vi "BinSearchVIhotcold.vi"(6 "RN":sgl, 8 "X0":sgl=0.5, 11 "Ring":i16(ring) items=["Cold", "Warm", "Hot"]) -> (3 "Xpot":sgl)   [LabVIEW 2019]
uses:
  <vilib>/Platform/TimedLoop/XDataNode/timing_clust.ctl
  <vilib>/Platform/TimedLoop/XDataNode/nitl_modes.ctl
  <vilib>/Platform/TimedLoop/XDataNode/wakeup.ctl
  <vilib>/rvi/Emulation/niFpgaGetClockAttributes.vi
  <vilib>/rvi/Emulation/niFpgaSctlEmulationGetInTimedLoop.vi
  <vilib>/rvi/Emulation/niFpgaEmulationReportErrorSimple.vi
  <vilib>/rvi/Emulation/niFpgaCriticalErrorInLSC.vi
  <vilib>/Platform/TimedLoop/XDataNode/XDataNode.xnode
  <vilib>/Platform/TimedLoop/XDataNode/XDNodeRunTimeDep.lvlib
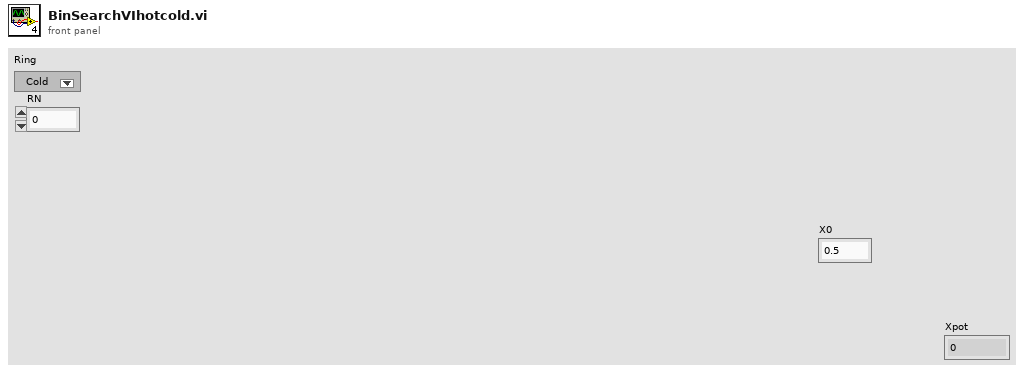
[diagram p1: front panel]
types:
  T1 = typedef "XDNodeRunTimeDep.lvlib/timing_clust.ctl" = cluster{"Expected End [f-1]":u64, "Actual End [f-1]":u64, "Finished Late? [f-1]":bool, "Expected End [i-1]":u64, "Actual End [i-1]":u64, "Finished Late? [i-1]":bool, "Expected Start [i]":u64, "Actual Start [i]":u64, "Expected Start [f]":u64, "Actual Start [f]":u64, "Source Name":string, "Structure Name":string, "Period":i64, "Deadline":i64, "Offset":i64, "Start":i64, "Priority":i32, "Timeout":i32, "Mode":T2, "Wakeup Reason":T3, "Error":errorcluster, "Source Type":string, "Secondary Source Type":string, "Global End Time":u64, "Global Start Time":u64, "Frame Duration":u64, "Iteration Duration":u64, "Assigned CPU":i32, "I/O Scan Engine Mode":u32}
  T2 = typedef "XDNodeRunTimeDep.lvlib/nitl_modes.ctl" = enum32{"No Change", "Process missed periods, maintain original phase", "Discard missed periods, maintain original phase", "Process missed periods, ignore original phase", "Discard missed periods, ignore original phase"}
  T3 = typedef "XDNodeRunTimeDep.lvlib/wakeup.ctl" = enum32{"Normal", "Aborted", "Asynchronous wakeup", "Timing source error", "Timed loop error", "Timeout"}
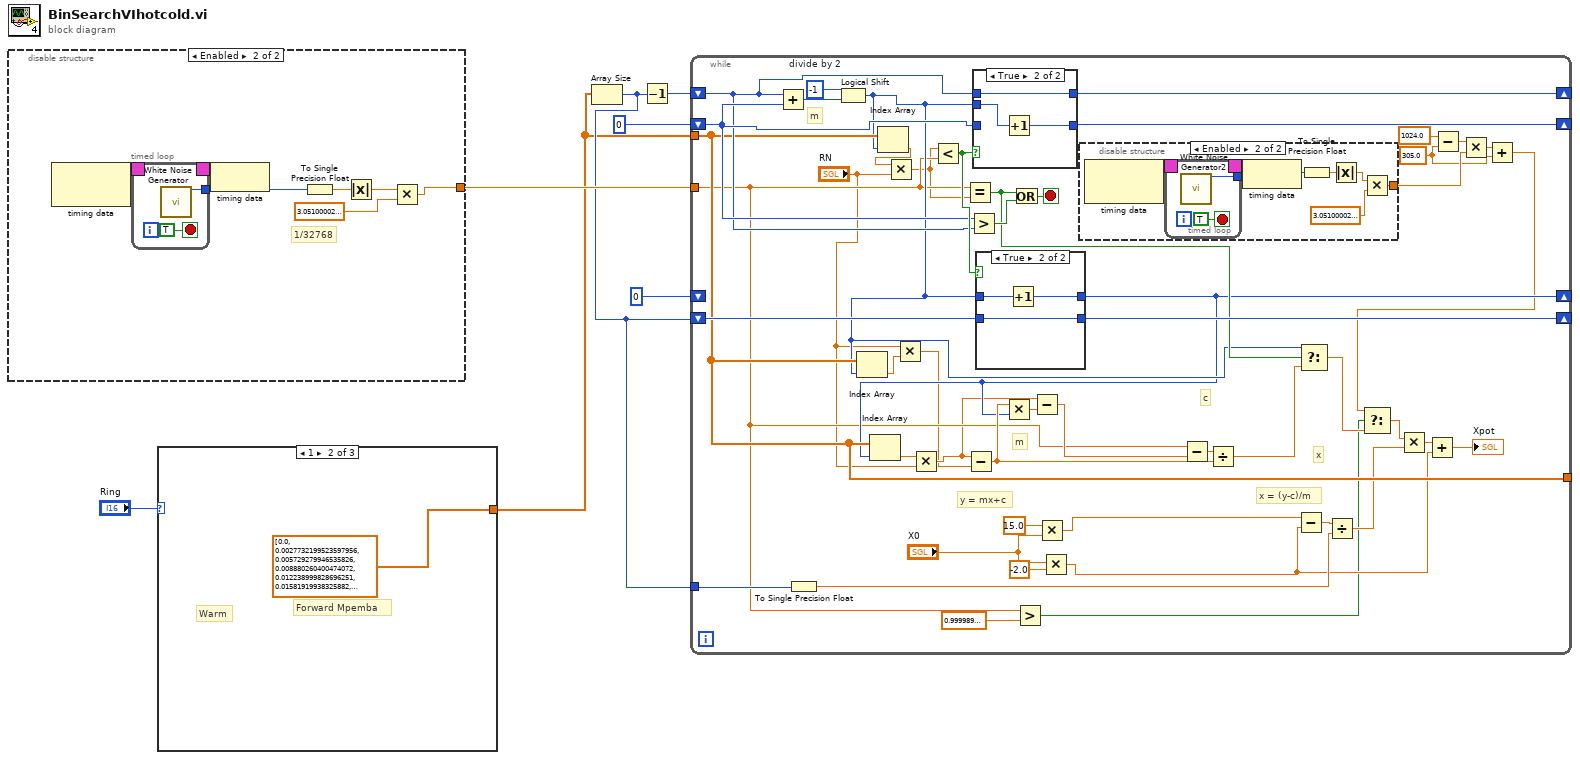
[diagram p0: block diagram]
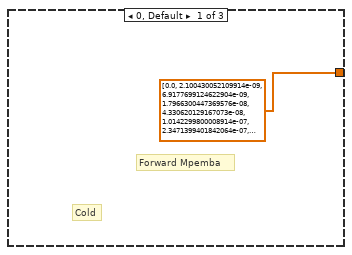
[diagram p2: hidden frame]
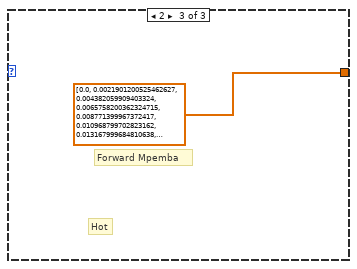
[diagram p3: hidden frame]
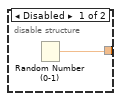
[diagram p4: hidden frame]
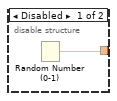
[diagram p5: hidden frame]
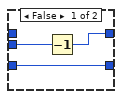
[diagram p7: hidden frame]
diagram:
  n1 = disable-structure shown="Enabled" {
    disable-tunnel: [w8 w11] -> w4
    frame Disabled {
      n2 = Random Number (0-1)() -> (number: 0 to 1=w8:dbl)
    }
    frame Enabled {
      # "1/32768"
      n3 = node-c288() -> (w10:T1)  [unwired: 1 in]
      n4 = timed-loop {
        timing: w10 -> [_]
        timing-out: [_] -> w9
        tunnel: [w17] -> w15
        stop <- TRUE stop-if-true
        n5 = call "White Noise Generator"() -> ("white noise out"=w17:i16)  [unwired: 15 in]
      }
      n6 = node-c288(w9) -> ()
      n7 = To Single Precision Float(number=w15) -> (single precision float=w13:sgl)
      n8 = Absolute Value(x=w13) -> (abs(x)=w12:sgl)
      n9 = Multiply(x=w12, y=sgl 3.051e-05) -> (x*y=w11:sgl)
    }
  }
  n10 = case shown="1" "Ring" {
    tunnel: [sgl[] [0.0, 2.10043e-09, 6.91777e-09, 1.79663e-08, 4.33062e-08, 1.01423e-07, 2.34714e-07, 5.40417e-07, 1.24154e-06, 2.84958e-06, 6.60417e-06, 1.50495e-05, 3.29051e-05, 6.8487e-05, 0.000135501, 0.0002551, 0.000457891, 0.000785411, 0.0012905, 0.00203611, 0.00309218, 0.00453075, 0.00641965, 0.00881572, 0.0117584, 0.0152648, 0.019327, 0.0239115, 0.0289619, 0.0344029, 0.0401462, 0.0460966, 0.0521583, 0.0582401, 0.0642597, 0.0701466, 0.0758436, 0.0813074, 0.0865076, 0.0914259, 0.0960546, 0.100394, 0.104453, 0.108243, 0.11178, 0.115085, 0.118176, 0.121075, 0.123802, 0.126379, 0.128825, 0.13116, 0.133402, 0.135569, 0.137679, 0.139748, 0.141793, 0.143832, 0.14588, 0.147957, 0.150081, 0.152272, 0.154553, 0.156947, 0.159484, 0.162193, 0.165111, 0.16828, 0.171747, 0.175568, 0.179807, 0.184542, 0.189859, 0.195861, 0.202666, 0.210409, 0.219246, 0.229351, 0.240917, 0.254157, 0.269299, 0.286581, 0.306242, 0.32851, 0.353589, 0.381636, 0.412741, 0.446898, 0.483987, 0.523744, 0.565749, 0.609418, 0.654015, 0.698674, 0.742448, 0.784365, 0.823503, 0.859064, 0.890444, 0.917278, 0.939468, 0.957175, 0.970777, 0.980814, 0.987911, 0.992708, 0.9958, 0.997696, 0.998798, 0.999405, 0.99972, 0.999874, 0.999945, 0.999976, 0.999989, 0.999995, 0.999998, 0.999999, 0.999999, 0.999999, 1.0, 1.0, 1.0, 1.0, 1.0, 1.0, 1.0, 1.0, 1.0, 1.0, 1.0, 1.0, 1.0, 1.0, 1.0, 1.0, 1.0, 1.0, 1.0, 1.0, 1.0, 1.0, 1.0, 1.0, 1.0, 1.0, 1.0, 1.0, 1.0, 1.0, 1.0, 1.0, 1.0, 1.0, 1.0, 1.0, 1.0, 1.0, 1.0, 1.0, 1.0, 1.0, 1.0, 1.0, 1.0, 1.0, 1.0, 1.0, 1.0, 1.0, 1.0, 1.0, 1.0, 1.0, 1.0, 1.0, 1.0, 1.0, 1.0, 1.0, 1.0, 1.0, 1.0, 1.0, 1.0, 1.0, 1.0, 1.0, 1.0, 1.0, 1.0, 1.0, 1.0, 1.0, 1.0, 1.0, 1.0, 1.0, 1.0, 1.0, 1.0, 1.0, 1.0, 1.0, 1.0, 1.0, 1.0, 1.0, 1.0, 1.0, 1.0, 1.0, 1.0, 1.0, 1.0, 1.0, 1.0, 1.0, 1.0, 1.0, 1.0, 1.0, 1.0, 1.0, 1.0, 1.0, 1.0, 1.0, 1.0, 1.0, 1.0, 1.0, 1.0, 1.0, 1.0, 1.0, 1.0, 1.0, 1.0, 1.0, 1.0, 1.0, 1.0, 1.0, 1.0, 1.0, 1.0, 1.0, 1.0, 1.0, 1.0, 1.0, 1.0, 1.0, 1.0, 1.0, 1.0, 1.0, 1.0, 1.0, 1.0, 1.0, 1.0, 1.0, 1.0, 1.0, 1.0, 1.0, 1.0, 1.0, 1.0, 1.0, 1.0, 1.0, 1.0, 1.0, 1.0, 1.0, 1.0, 1.0, 1.0, 1.0, 1.0, 1.0, 1.0, 1.0, 1.0, 1.0, 1.0, 1.0, 1.0, 1.0, 1.0, 1.0, 1.0, 1.0, 1.0, 1.0, 1.0, 1.0, 1.0, 1.0, 1.0, 1.0, 1.0, 1.0, 1.0, 1.0, 1.0, 1.0, 1.0, 1.0, 1.0, 1.0, 1.0, 1.0, 1.0, 1.0, 1.0, 1.0, 1.0, 1.0, 1.0, 1.0, 1.0, 1.0, 1.0, 1.0, 1.0, 1.0, 1.0, 1.0, 1.0, 1.0, 1.0, 1.0, 1.0, 1.0, 1.0, 1.0, 1.0, 1.0, 1.0, 1.0, 1.0, 1.0, 1.0, 1.0, 1.0, 1.0, 1.0, 1.0, 1.0, 1.0, 1.0, 1.0, 1.0, 1.0, 1.0, 1.0, 1.0, 1.0, 1.0, 1.0, 1.0, 1.0, 1.0, 1.0, 1.0, 1.0, 1.0, 1.0, 1.0, 1.0, 1.0, 1.0, 1.0, 1.0, 1.0, 1.0, 1.0, 1.0, 1.0, 1.0, 1.0, 1.0, 1.0, 1.0, 1.0, 1.0, 1.0, 1.0, 1.0, 1.0, 1.0, 1.0, 1.0, 1.0, 1.0, 1.0, 1.0, 1.0, 1.0, 1.0, 1.0, 1.0, 1.0, 1.0, 1.0, 1.0, 1.0, 1.0, 1.0, 1.0, 1.0, 1.0, 1.0, 1.0, 1.0, 1.0, 1.0, 1.0, 1.0, 1.0, 1.0, 1.0, 1.0, 1.0, 1.0, 1.0, 1.0, 1.0, 1.0, 1.0, 1.0, 1.0, 1.0, 1.0, 1.0, 1.0, 1.0, 1.0, 1.0, 1.0, 1.0, 1.0, 1.0, 1.0, 1.0, 1.0, 1.0, 1.0, 1.0, 1.0, 1.0, 1.0, 1.0, 1.0, 1.0, 1.0, 1.0, 1.0, 1.0, 1.0, 1.0, 1.0, 1.0, 1.0, 1.0, 1.0, 1.0, 1.0, 1.0, 1.0, 1.0, 1.0, 1.0, 1.0, 1.0, 1.0, 1.0, 1.0, 1.0, 1.0, 1.0, 1.0, 1.0, 1.0, 1.0, 1.0, 1.0, 1.0, 1.0, 1.0, 1.0, 1.0, 1.0, 1.0, 1.0, 1.0, 1.0, 1.0, 1.0, 1.0, 1.0, 1.0, 1.0, 1.0, 1.0, 1.0, 1.0, 1.0] ("Init Data Out") sgl[] [0.0, 0.00277322, 0.00572928, 0.00888026, 0.012239, 0.0158192, 0.0196354, 0.0237033, 0.0280394, 0.0326614, 0.0375931, 0.0428469, 0.0484165, 0.0542936, 0.0604679, 0.0669269, 0.0736569, 0.0806426, 0.0878674, 0.0953142, 0.102965, 0.110802, 0.118805, 0.126958, 0.135242, 0.143639, 0.152132, 0.160705, 0.169342, 0.178029, 0.186753, 0.1955, 0.20426, 0.213023, 0.221778, 0.230518, 0.239236, 0.247927, 0.256584, 0.265204, 0.273784, 0.282321, 0.290814, 0.299263, 0.307668, 0.316028, 0.324345, 0.332622, 0.34086, 0.349062, 0.357231, 0.365371, 0.373486, 0.381579, 0.389656, 0.397721, 0.405778, 0.413834, 0.421893, 0.42996, 0.438041, 0.446141, 0.454267, 0.462422, 0.470614, 0.478848, 0.487129, 0.495462, 0.503852, 0.512306, 0.520828, 0.529422, 0.538093, 0.546845, 0.555682, 0.564607, 0.573624, 0.582733, 0.591938, 0.60124, 0.610637, 0.620131, 0.629719, 0.6394, 0.64917, 0.659025, 0.668958, 0.678964, 0.689033, 0.699156, 0.709323, 0.71952, 0.729733, 0.739948, 0.750147, 0.760311, 0.770422, 0.780458, 0.790398, 0.800217, 0.809893, 0.819401, 0.828716, 0.837814, 0.84667, 0.85526, 0.863562, 0.871554, 0.879215, 0.886528, 0.893477, 0.900049, 0.906232, 0.912032, 0.917473, 0.922578, 0.927367, 0.93186, 0.936075, 0.940029, 0.943739, 0.947219, 0.950484, 0.953547, 0.95642, 0.959116, 0.961645, 0.964018, 0.966243, 0.968332, 0.97029, 0.972128, 0.973852, 0.97547, 0.976987, 0.978411, 0.979746, 0.980999, 0.982175, 0.983277, 0.984312, 0.985282, 0.986193, 0.987047, 0.987848, 0.9886, 0.989305, 0.989967, 0.990587, 0.99117, 0.991716, 0.992228, 0.992709, 0.99316, 0.993583, 0.99398, 0.994353, 0.994702, 0.99503, 0.995337, 0.995626, 0.995897, 0.99615, 0.996389, 0.996612, 0.996822, 0.997018, 0.997203, 0.997376, 0.997538, 0.997691, 0.997834, 0.997968, 0.998093, 0.998211, 0.998322, 0.998426, 0.998523, 0.998615, 0.9987, 0.998781, 0.998856, 0.998927, 0.998994, 0.999056, 0.999114, 0.999169, 0.999221, 0.999269, 0.999314, 0.999357, 0.999397, 0.999434, 0.999469, 0.999502, 0.999533, 0.999562, 0.999589, 0.999614, 0.999638, 0.999661, 0.999682, 0.999702, 0.99972, 0.999738, 0.999754, 0.999769, 0.999783, 0.999797, 0.99981, 0.999821, 0.999833, 0.999843, 0.999853, 0.999862, 0.99987, 0.999879, 0.999886, 0.999893, 0.9999, 0.999906, 0.999912, 0.999917, 0.999923, 0.999927, 0.999932, 0.999936, 0.99994, 0.999944, 0.999948, 0.999951, 0.999954, 0.999957, 0.99996, 0.999962, 0.999965, 0.999967, 0.999969, 0.999971, 0.999973, 0.999974, 0.999976, 0.999978, 0.999979, 0.99998, 0.999982, 0.999983, 0.999984, 0.999985, 0.999986, 0.999987, 0.999988, 0.999989, 0.999989, 0.99999, 0.999991, 0.999991, 0.999992, 0.999992, 0.999993, 0.999994, 0.999994, 0.999994, 0.999995, 0.999995, 0.999996, 0.999996, 0.999996, 0.999996, 0.999997, 0.999997, 0.999997, 0.999997, 0.999998, 0.999998, 0.999998, 0.999998, 0.999998, 0.999999, 0.999999, 0.999999, 0.999999, 0.999999, 0.999999, 0.999999, 0.999999, 1.0, 1.0, 1.0, 1.0, 1.0, 1.0, 1.0, 1.0, 1.0, 1.0, 1.0, 1.0, 1.0, 1.0, 1.0, 1.0, 1.0, 1.0, 1.0, 1.0, 1.0, 1.0, 1.0, 1.0, 1.0, 1.0, 1.0, 1.0, 1.0, 1.0, 1.0, 1.0, 1.0, 1.0, 1.0, 1.0, 1.0, 1.0, 1.0, 1.0, 1.0, 1.0, 1.0, 1.0, 1.0, 1.0, 1.0, 1.0, 1.0, 1.0, 1.0, 1.0, 1.0, 1.0, 1.0, 1.0, 1.0, 1.0, 1.0, 1.0, 1.0, 1.0, 1.0, 1.0, 1.0, 1.0, 1.0, 1.0, 1.0, 1.0, 1.0, 1.0, 1.0, 1.0, 1.0, 1.0, 1.0, 1.0, 1.0, 1.0, 1.0, 1.0, 1.0, 1.0, 1.0, 1.0, 1.0, 1.0, 1.0, 1.0, 1.0, 1.0, 1.0, 1.0, 1.0, 1.0, 1.0, 1.0, 1.0, 1.0, 1.0, 1.0, 1.0, 1.0, 1.0, 1.0, 1.0, 1.0, 1.0, 1.0, 1.0, 1.0, 1.0, 1.0, 1.0, 1.0, 1.0, 1.0, 1.0, 1.0, 1.0, 1.0, 1.0, 1.0, 1.0, 1.0, 1.0, 1.0, 1.0, 1.0, 1.0, 1.0, 1.0, 1.0, 1.0, 1.0, 1.0, 1.0, 1.0, 1.0, 1.0, 1.0, 1.0, 1.0, 1.0, 1.0, 1.0, 1.0, 1.0, 1.0, 1.0, 1.0, 1.0, 1.0, 1.0, 1.0, 1.0, 1.0, 1.0, 1.0, 1.0, 1.0, 1.0, 1.0, 1.0, 1.0, 1.0, 1.0, 1.0, 1.0, 1.0, 1.0, 1.0, 1.0, 1.0, 1.0, 1.0, 1.0, 1.0, 1.0, 1.0, 1.0, 1.0, 1.0, 1.0, 1.0, 1.0, 1.0, 1.0, 1.0, 1.0, 1.0, 1.0, 1.0, 1.0, 1.0, 1.0, 1.0, 1.0, 1.0, 1.0, 1.0, 1.0, 1.0, 1.0, 1.0, 1.0, 1.0, 1.0, 1.0, 1.0, 1.0, 1.0, 1.0, 1.0, 1.0, 1.0, 1.0, 1.0, 1.0, 1.0, 1.0, 1.0, 1.0, 1.0, 1.0] ("Init Data Out") sgl[] [0.0, 0.00219012, 0.00438206, 0.00657582, 0.0087714, 0.0109688, 0.013168, 0.0153691, 0.017572, 0.0197767, 0.0219833, 0.0241916, 0.0264017, 0.0286133, 0.0308264, 0.0330407, 0.0352562, 0.0374728, 0.0396904, 0.0419088, 0.044128, 0.0463479, 0.0485685, 0.0507895, 0.053011, 0.0552329, 0.0574552, 0.0596777, 0.0619004, 0.0641233, 0.0663463, 0.0685694, 0.0707925, 0.0730156, 0.0752387, 0.0774618, 0.0796848, 0.0819077, 0.0841305, 0.0863532, 0.0885757, 0.0907981, 0.0930203, 0.0952424, 0.0974643, 0.0996861, 0.101908, 0.104129, 0.106351, 0.108572, 0.110793, 0.113014, 0.115235, 0.117456, 0.119676, 0.121897, 0.124118, 0.126339, 0.128559, 0.13078, 0.133001, 0.135222, 0.137443, 0.139664, 0.141885, 0.144106, 0.146328, 0.14855, 0.150771, 0.152994, 0.155216, 0.157438, 0.159661, 0.161884, 0.164108, 0.166331, 0.168555, 0.17078, 0.173004, 0.175229, 0.177454, 0.17968, 0.181905, 0.184131, 0.186358, 0.188584, 0.190811, 0.193038, 0.195265, 0.197492, 0.19972, 0.201947, 0.204175, 0.206403, 0.20863, 0.210858, 0.213085, 0.215312, 0.217539, 0.219765, 0.221991, 0.224217, 0.226442, 0.228666, 0.230889, 0.233112, 0.235333, 0.237554, 0.239773, 0.241991, 0.244207, 0.246422, 0.248635, 0.250847, 0.253056, 0.255264, 0.257469, 0.259673, 0.261875, 0.264075, 0.266274, 0.26847, 0.270665, 0.272858, 0.275049, 0.277239, 0.279426, 0.281612, 0.283796, 0.285978, 0.288158, 0.290336, 0.292513, 0.294688, 0.296861, 0.299032, 0.301201, 0.303369, 0.305535, 0.307699, 0.309861, 0.312022, 0.31418, 0.316337, 0.318492, 0.320645, 0.322797, 0.324947, 0.327095, 0.329241, 0.331385, 0.333528, 0.335668, 0.337807, 0.339945, 0.34208, 0.344214, 0.346346, 0.348476, 0.350604, 0.352731, 0.354856, 0.356979, 0.3591, 0.36122, 0.363338, 0.365454, 0.367568, 0.36968, 0.371791, 0.3739, 0.376008, 0.378113, 0.380217, 0.382319, 0.384419, 0.386518, 0.388615, 0.39071, 0.392803, 0.394895, 0.396985, 0.399073, 0.401159, 0.403244, 0.405327, 0.407408, 0.409487, 0.411565, 0.413641, 0.415716, 0.417788, 0.419859, 0.421928, 0.423996, 0.426061, 0.428125, 0.430188, 0.432248, 0.434307, 0.436364, 0.43842, 0.440474, 0.442526, 0.444576, 0.446625, 0.448672, 0.450717, 0.45276, 0.454802, 0.456842, 0.458881, 0.460918, 0.462953, 0.464986, 0.467018, 0.469048, 0.471076, 0.473103, 0.475128, 0.477151, 0.479173, 0.481193, 0.483211, 0.485228, 0.487243, 0.489256, 0.491267, 0.493277, 0.495285, 0.497292, 0.499297, 0.5013, 0.503302, 0.505302, 0.5073, 0.509297, 0.511292, 0.513285, 0.515276, 0.517266, 0.519255, 0.521241, 0.523226, 0.52521, 0.527192, 0.529172, 0.53115, 0.533127, 0.535102, 0.537076, 0.539048, 0.541018, 0.542987, 0.544954, 0.546919, 0.548883, 0.550845, 0.552805, 0.554764, 0.556721, 0.558677, 0.560631, 0.562583, 0.564534, 0.566483, 0.568431, 0.570377, 0.572321, 0.574263, 0.576204, 0.578144, 0.580082, 0.582018, 0.583952, 0.585885, 0.587817, 0.589747, 0.591675, 0.593602, 0.595527, 0.59745, 0.599372, 0.601292, 0.603211, 0.605128, 0.607043, 0.608957, 0.610869, 0.61278, 0.614689, 0.616596, 0.618502, 0.620407, 0.622309, 0.624211, 0.62611, 0.628008, 0.629905, 0.6318, 0.633693, 0.635585, 0.637475, 0.639363, 0.64125, 0.643136, 0.64502, 0.646902, 0.648783, 0.650662, 0.65254, 0.654416, 0.65629, 0.658163, 0.660035, 0.661905, 0.663773, 0.66564, 0.667505, 0.669369, 0.671231, 0.673091, 0.67495, 0.676808, 0.678664, 0.680518, 0.682371, 0.684223, 0.686072, 0.687921, 0.689767, 0.691613, 0.693456, 0.695298, 0.697139, 0.698978, 0.700816, 0.702652, 0.704486, 0.706319, 0.708151, 0.709981, 0.711809, 0.713636, 0.715461, 0.717285, 0.719108, 0.720929, 0.722748, 0.724566, 0.726382, 0.728197, 0.73001, 0.731822, 0.733632, 0.735441, 0.737248, 0.739054, 0.740859, 0.742661, 0.744463, 0.746262, 0.748061, 0.749858, 0.751653, 0.753447, 0.755239, 0.75703, 0.75882, 0.760607, 0.762394, 0.764179, 0.765962, 0.767744, 0.769525, 0.771304, 0.773081, 0.774857, 0.776632, 0.778405, 0.780177, 0.781947, 0.783716, 0.785483, 0.787249, 0.789013, 0.790776, 0.792537, 0.794297, 0.796056, 0.797813, 0.799568, 0.801322, 0.803075, 0.804826, 0.806576, 0.808324, 0.810071, 0.811817, 0.81356, 0.815303, 0.817044, 0.818784, 0.820522, 0.822258, 0.823994, 0.825728, 0.82746, 0.829191, 0.83092, 0.832649, 0.834375, 0.8361, 0.837824, 0.839547, 0.841267, 0.842987, 0.844705, 0.846422, 0.848137, 0.849851, 0.851563, 0.853274, 0.854984, 0.856692, 0.858398, 0.860104, 0.861808, 0.86351, 0.865211, 0.866911, 0.868609, 0.870306, 0.872001, 0.873695, 0.875388, 0.877079, 0.878769, 0.880457, 0.882144, 0.88383, 0.885514, 0.887197, 0.888878, 0.890558, 0.892237, 0.893914, 0.89559, 0.897264, 0.898937, 0.900609, 0.902279, 0.903948, 0.905616, 0.907282, 0.908946, 0.91061, 0.912272, 0.913932, 0.915592, 0.917249, 0.918906, 0.920561, 0.922215, 0.923867, 0.925518, 0.927168, 0.928816, 0.930463, 0.932108, 0.933752, 0.935395, 0.937037, 0.938677, 0.940315, 0.941953, 0.943589, 0.945223, 0.946856, 0.948488, 0.950119, 0.951748, 0.953376, 0.955002, 0.956627, 0.958251, 0.959874, 0.961495, 0.963115, 0.964733, 0.96635, 0.967966, 0.96958, 0.971193, 0.972805, 0.974415, 0.976024, 0.977632, 0.979238, 0.980843, 0.982447, 0.984049, 0.98565, 0.98725, 0.988849, 0.990446, 0.992041, 0.993636, 0.995229, 0.996821, 0.998411, 1.0] ("Init Data Out")] -> w1
    frame 0, Default {
      # "Forward Mpemba"
      # "Cold"
    }
    frame 1 {
      # "Forward Mpemba"
      # "Warm"
    }
    frame 2 {
      # "Forward Mpemba"
      # "Hot"
    }
  }
  n11 = Array Size(array=w1) -> (size(s)=w3:i32)
  n12 = Decrement(x=w3) -> (x-1=w5:i32)
  n13 = while {
    tunnel: w1 -> [w62]
    tunnel: w4 -> [w42]
    shift-right: [w72] -> _
    shift-left: w5 -> [w63]
    shift-right: [w68] -> _
    shift-left: 0 -> [w64]
    shift-right: [w54] -> _
    shift-left: 0 -> [_]
    shift-right: [w65] -> _
    shift-left: w3 -> [w66]
    tunnel: [w62] -> _
    tunnel: w3 -> [w48]
    stop <- w70 stop-if-true
    w35 = sgl 305.0 ("y")
    w73 = -1  # divide by 2
    # "x"
    # "x = (y-c)/m"
    # "c"
    # "m"
    # "y = mx+c"
    # "m"
    n14 = Add(x=w63, y=w64) -> (x+y=w69:i32)
    n15 = To Single Precision Float(number=w48) -> (single precision float=w47:sgl)
    n16 = Logical Shift(y=w73, x=w69) -> (x << y=w60:i32)
    n17 = Index Array(array=w62, index=w60) -> (element=w27:sgl)
    n18 = Index Array(array=w62, index=w60) -> (element=w31:sgl)
    n19 = Multiply(x=w31, y="RN") -> (x*y=w30:sgl)
    n20 = Multiply(x="RN", y=w27) -> (x*y=w25:sgl)
    n21 = Less?(x=w30, y=w42) -> (x < y?=w67:bool)
    n22 = Equal?(x=w42, y=w30) -> (x = y?=w61:bool)
    n23 = Greater?(x=w64, y=w63) -> (0:w71:bool)
    n24 = case shown="True" w67 {
      tunnel: w60 -> [w95 w98]
      tunnel: [w94 w96] -> w72
      tunnel: w64 -> [w93 _]
      tunnel: [w93 w97] -> w68
      tunnel: w63 -> [_ w96]
      frame False {
        n25 = Decrement(x=w95) -> (x-1=w94:i32)
      }
      frame True {
        n26 = Increment(x=w98) -> (x+1=w97:i32)
      }
    }
    n27 = case shown="True" w67 {
      tunnel: w60 -> [w89 w92]
      tunnel: [w88 w91] -> w54
      tunnel: w66 -> [w88 w90]
      tunnel: [w89 w90] -> w65
      frame False {
      }
      frame True {
        n28 = Increment(x=w92) -> (x+1=w91:i32)
      }
    }
    n29 = Index Array(array=w62, index=w54) -> (element=w29:sgl)
    n30 = Multiply(x=w29, y="RN") -> (x*y=w28:sgl)
    n31 = Subtract(x=w28, y=w25) -> (x-y=w56:sgl)
    n32 = Multiply(x=w56, y=w54) -> (x*y=w59:sgl)
    n33 = Or(x=w61, y=w71) -> (x .or. y?=w70:bool)
    n34 = Greater?(x=w42, y=sgl 0.99999) -> (0:w32:bool)
    n35 = Subtract(x=w28, y=w59) -> (x-y=w58:sgl)
    n36 = Multiply(x=sgl 15.0, y="X0") -> (x*y=w51:sgl)
    n37 = Multiply(x="X0", y=sgl -2.0) -> (x*y=w45:sgl)
    n38 = disable-structure shown="Enabled" {
      disable-tunnel: [w74 w77] -> w37
      frame Disabled {
        n39 = Random Number (0-1)() -> (number: 0 to 1=w74:dbl)
      }
      frame Enabled {
        n40 = node-c288() -> (w76:T1)  [unwired: 1 in]
        n41 = timed-loop {
          timing: w76 -> [_]
          timing-out: [_] -> w75
          tunnel: [w83] -> w81
          stop <- TRUE stop-if-true
          n42 = call "White Noise Generator2"() -> ("white noise out"=w83:i16)  [unwired: 15 in]
        }
        n43 = node-c288(w75) -> ()
        n44 = To Single Precision Float(number=w81) -> (single precision float=w79:sgl)
        n45 = Absolute Value(x=w79) -> (abs(x)=w78:sgl)
        n46 = Multiply(x=w78, y=sgl 3.051e-05) -> (x*y=w77:sgl)
      }
    }
    n47 = Subtract(x=w42, y=w58) -> (x-y=w57:sgl)
    n48 = Divide(x=w57, y=w56) -> (x/y=w55:sgl)
    n49 = Subtract(x=w51, y=w45) -> (x-y=w50:sgl)
    n50 = Select(t=w60, s=w61, f=w55) -> (s? t:f=w40:sgl)
    n51 = Divide(x=w50, y=w47) -> (x/y=w49:sgl)
    n52 = Subtract(x=sgl 1024.0, y=w35) -> (x-y=w38:sgl)
    n53 = Multiply(x=w38, y=w37) -> (x*y=w36:sgl)
    n54 = Add(x=w36, y=w35) -> (x+y=w33:sgl)
    n55 = Select(t=w33, s=w32, f=w40) -> (s? t:f=w34:sgl)
    n56 = Multiply(x=w34, y=w49) -> (x*y=w46:sgl)
    n57 = Add(x=w46, y=w45) -> (x+y=→"Xpot":sgl)
  }
